vi "gps.vi"(0 "纬度":string, 1 "经度":string, 2 "滑动杆":i16(slide) scale=3.5..18.0, 3 "地图":refnum<k7>(container) caption="网页浏览器", 4 "error IO":errorcluster) -> (5 "错误输出":errorcluster)   [LabVIEW 2018]
panel:
  out "转换后纬度":string
  out "转换后经度":string
  out "状态显示":string
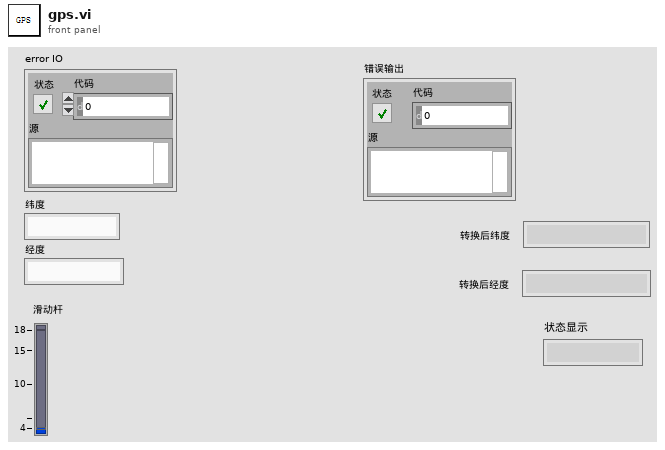
[diagram p1: front panel]
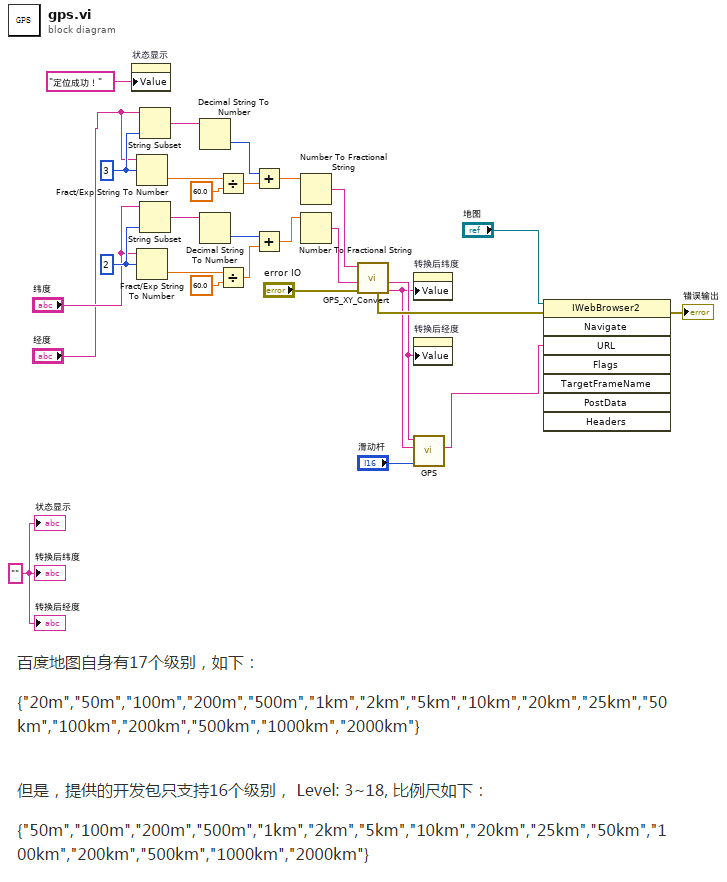
[diagram p0: block diagram]
diagram:
  w10 = 2 ("整数部分长度 2")
  w18 = 3 ("整数部分长度")
  w28 = ""
  n1 = property on="状态显示" class="Str"("Value"="定位成功！") -> ()  [unwired: 2 in, 2 out]
  n2 = Fract/Exp String To Number(string="经度", offset=w18) -> (number=w13:dbl)  [unwired: 2 in, 1 out]
  n3 = Fract/Exp String To Number(string="纬度", offset=w10) -> (number=w5:dbl)  [unwired: 2 in, 1 out]
  n4 = String Subset(string="经度", length (rest)=w18) -> (substring=w12:string)  [unwired: 1 in]
  n5 = String Subset(string="纬度", length (rest)=w10) -> (substring=w4:string)  [unwired: 1 in]
  n6 = Decimal String To Number(string=w12) -> (number=w15:i32)  [unwired: 2 in, 1 out]
  n7 = Decimal String To Number(string=w4) -> (number=w7:i32)  [unwired: 2 in, 1 out]
  n8 = Divide(x=w13, y=60.0) -> (x/y=w16:dbl)
  n9 = Divide(x=w5, y=60.0) -> (x/y=w8:dbl)
  n10 = Add(x=w15, y=w16) -> (x+y=w17:dbl)
  n11 = Add(x=w7, y=w8) -> (x+y=w9:dbl)
  n12 = Number To Fractional String(number=w17) -> (F-format string=w11:string)  [unwired: 3 in]
  n13 = Number To Fractional String(number=w9) -> (F-format string=w3:string)  [unwired: 3 in]
  n14 = call "GPS_XY_Convert.vi"("error in (no error)"="error IO", "纬度"=w3, "经度"=w11) -> ("转换之后的纬度2"=w21:string, "转换之后的经度2"=w22:string, "error out"=w26:errorcluster)  [unwired: 4 in, 2 out]
  n15 = property on="转换后纬度" class="Str"("Value"=w21) -> ()  [unwired: 2 in, 2 out]
  n16 = property on="转换后经度" class="Str"("Value"=w22) -> ()  [unwired: 2 in, 2 out]
  n17 = call "GPS .vi"("滑动杆"="滑动杆", "纬度"=w21, "经度"=w22) -> ("url"=w25:string)  [unwired: 8 in]
  n18 = invoke class="IWebBrowser2" method="Navigate"(reference="地图", error in=w26, "URL"=w25) -> (error out=→"错误输出":errorcluster)  [unwired: 5 in, 7 out]
  "转换后经度" <- w28
  "转换后纬度" <- w28
  "状态显示" <- w28
